vi "Decode response.vi"(8 "error in (no error)":errorcluster, 10 "Recieved":string, 11 "Command":string) -> (0 "error out":errorcluster, 2 "Command Accepted":bool, 3 "Remainning response":string)   [LabVIEW 2024, in "RSeries_CAM.lvlib" / "RSeries_CAM.lvclass"]
uses:
  RSeries_CAM.lvclass
panel:
  out "output 3":string
  out "remaining string":string
  out "output 2":i32
  out "output 1":string
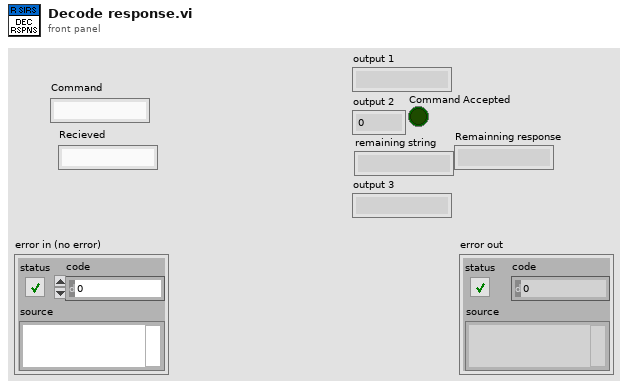
[diagram p1: front panel]
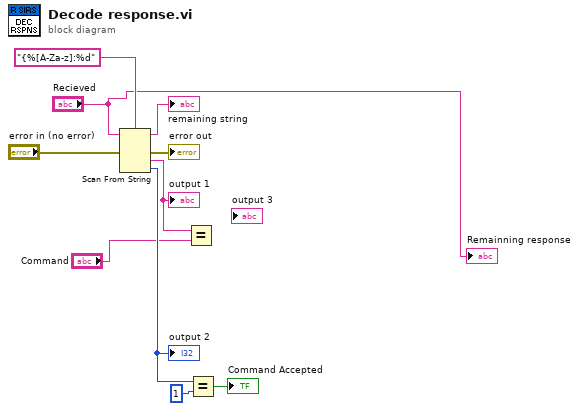
[diagram p0: block diagram]
diagram:
  n1 = Scan From String(format string="{%[A-Za-z]:%d", input string="Recieved", error in="error in (no error)") -> (remaining string=→"remaining string":string, error out=→"error out":errorcluster, output 1=w3:string, output 2=w9:i32)  [unwired: 3 in, 1 out]
  "output 1" <- w3
  "output 2" <- w9
  n2 = Equal?(x=w3, y="Command") -> ()  [unwired: 1 out]
  n3 = Equal?(x=w9, y=1) -> (x = y?=→"Command Accepted":bool)
  "Remainning response" <- "Recieved"
